vi "Drive Global Data.vi"() -> ()   [LabVIEW 2012]
panel:
  in  "X All Power?":bool
  in  "Wanted dead band value":dbl
  in  "Driver JoyStick Info":cluster{"Slow Drive?":bool, "Axisses":dbl[]}
  # "X"
  # "Y"
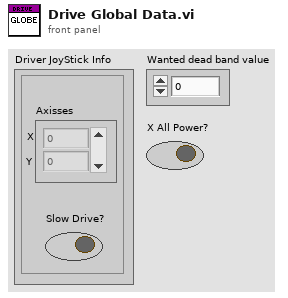
[diagram p1: front panel]
diagram:
